vi "Pass VI Ref.vi"(8 "error in (no error)":errorcluster, 9 "Name in":string, 10 "VI Ref in":refnum<vi>, 11 "View Interface in":refnum<class "Controller Actor.lvclass">) -> (0 "error out":errorcluster, 3 "View Interface out":refnum<class "Controller Actor.lvclass">)   [LabVIEW 2023, in "Event Actors.lvlib" / "Controller Actor.lvclass"]
uses:
  Controller Actor.lvclass
  Controller Actor.lvclass/Controller Actor.ctl
  Hardware Controller/Source/LSI Hardware Controller/IView Messages/Pass VI Ref Msg/Pass VI Ref Msg.lvclass
  <vilib>/ActorFramework/Actor/Actor.lvclass
  C:/Program Files/National Instruments/LabVIEW 2023/vi.lib/MGI/Monitored Actor/Monitored Actor/Monitored Actor/Monitored Actor.lvclass
  C:/Program Files/National Instruments/LabVIEW 2023/vi.lib/ActorFramework/Actor/Actor.lvclass
  C:/Projects/Shared Libraries/Event Actors/Controller Actor/Controller Actor.lvclass
  C:/Projects/Hardware Controller/Source/LSI Hardware Controller/View Interface/IView.lvclass
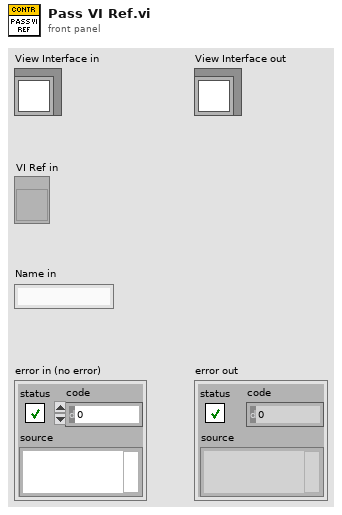
[diagram p1: front panel]
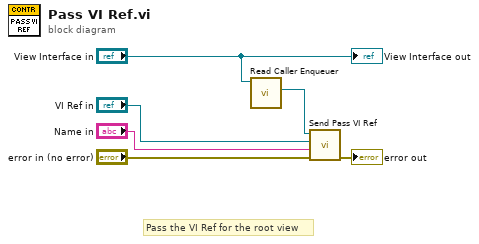
[diagram p0: block diagram]
diagram:
  # "Pass the VI Ref for the root view"
  n1 = call <vilib>:"Read Caller Enqueuer.vi"("Actor"="View Interface in") -> ("Caller Enqueuer"=w6:refnum<class "Message Enqueuer.lvclass">)  [unwired: 10 in]
  n2 = call "Send Pass VI Ref.vi"("error in (no error)"="error in (no error)", "Name in"="Name in", "VI Ref in"="VI Ref in", "Message Enqueuer"=w6) -> ("error out"=→"error out":errorcluster)  [unwired: 6 in, 1 out]
  "View Interface out" <- "View Interface in"
